vi "Iterator Enqueue.vi"(8 "error in (no error)":errorcluster, 10 "Iterator":refnum<class "Iterator.lvclass">, 11 "CompositeIterator in":refnum<class "CompositeIterator.lvclass">) -> (0 "error out":errorcluster, 3 "CompositeIterator out":refnum<class "CompositeIterator.lvclass">)   [LabVIEW 2015, in "CompositeIterator.lvclass"]
uses:
  CompositeIterator.lvclass
  Interface/Iterator.lvclass
  CompositeIterator.lvclass/CompositeIterator.ctl
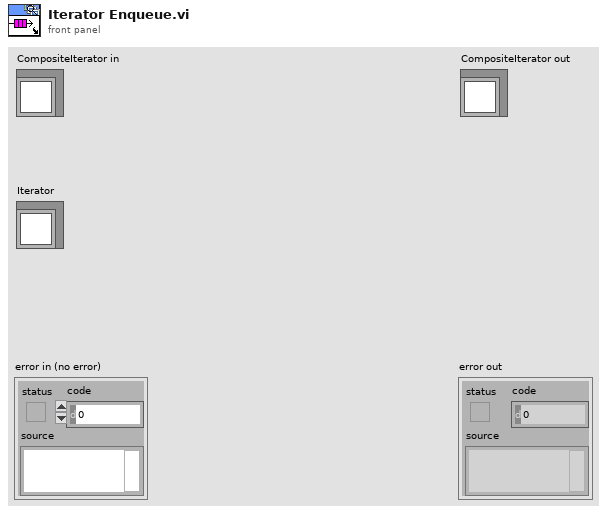
[diagram p1: front panel]
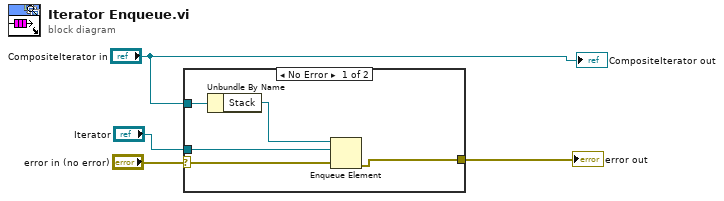
[diagram p0: block diagram]
diagram:
  n1 = case shown="No Error" "error in (no error)" {
    selector: "error in (no error)" -> [w7 w10]
    tunnel: "Iterator" -> [w8 _]
    tunnel: "CompositeIterator in" -> [w6 _]
    tunnel: [w5 w10] -> w1
    frame No Error {
      n2 = Unbundle By Name(w6) -> ("Stack"=w9:refnum<queue>)
      n3 = Enqueue Element(queue=w9, element=w8, error in (no error)=w7) -> (error out=w5:errorcluster)  [unwired: 1 in, 2 out]
    }
    frame Error {
    }
  }
  "error out" <- w1
  "CompositeIterator out" <- "CompositeIterator in"
